vi "Measure Voltage.vi"(7 "Channel List (101:110)":string="101:110", 8 "error in (no error)":errorcluster, 10 "Sample Count":i32=1, 11 "VISA resource name":refnum<visa-resource-name>="COM15") -> (0 "error out":errorcluster, 2 "Voltage Data":dbl[](array[numeric])=[-0.0818253011], 3 "Voltage":dbl=-0.0818253011 format="%0.8f")   [LabVIEW 2015]
uses:
  <instrlib>/Keithley 27XX/Public/Data/Read Multiple Direct.vi
  <instrlib>/Keithley 27XX/Keithley 27XX.lvlib
panel:
  in  "Serial Configuration":T1={"Baud Rate (19200)"=19200, "Flow Control (1: XON/XOFF)"=1, "Termination Char (0:CR)"=0} {"Termination Char (0:CR)" items=["CR", "LF"]; "Flow Control (1: XON/XOFF)" items=["None", "XON/XOFF", "RTS/CTS (2701 Only)", "XON/XOFF & RTS/CTS (2701 Only)"]; "Baud Rate (19200)" items=["300"=300, "600"=600, "1200"=1200, "2400"=2400, "4800"=4800, "9600"=9600, "19.2k"=19200, "38.4k (2701 Only)"=38400, "57.6k (2701 Only)"=57600, "115.2k (2701 Only)"=115200]}
  in  "Timeout (5000 milliseconds)":u32=5000
  in  "Function (0: DC Voltage)":u16(ring) items=["DC Voltage", "AC Voltage", "DC Current", "AC Current", "Resistance", "Four-Wire Resistance", "Temperature (C)", "Frequency", "Period", "Continuity"]
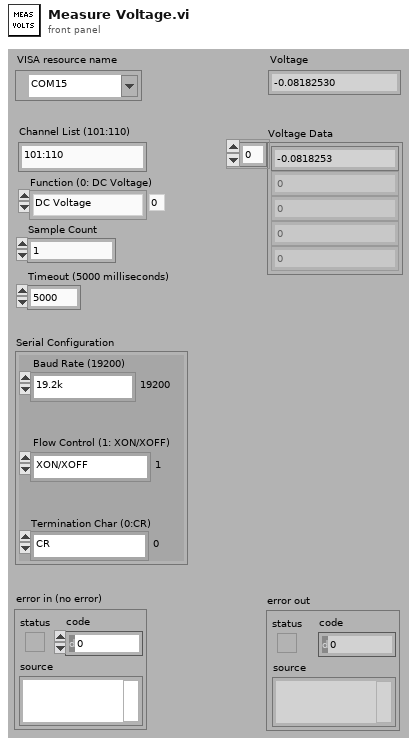
[diagram p1: front panel]
types:
  T1 = cluster{"Baud Rate (19200)":u32, "Flow Control (1: XON/XOFF)":u16, "Termination Char (0:CR)":u16}
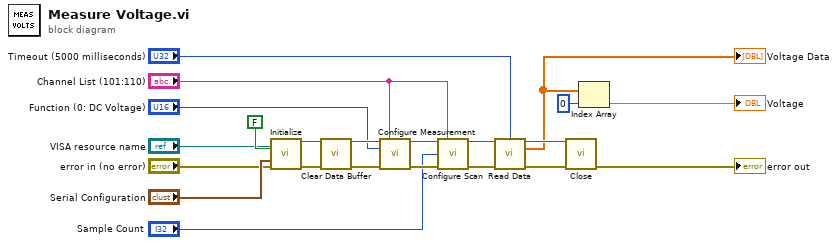
[diagram p0: block diagram]
diagram:
  n1 = call <instrlib>:"Initialize.vi"("VISA resource name"="VISA resource name", "ID Query? (T: Yes)"=FALSE, "Serial Configuration"="Serial Configuration", "error in (no error)"="error in (no error)") -> ("VISA resource name out"=w15:refnum<visa-resource-name>, "error out"=w16:errorcluster)  [unwired: 10 in]
  n2 = call <instrlib>:"Clear Data Buffer.vi"("VISA resource name"=w15, "error in (no error)"=w16) -> ("VISA resource name out"=w18:refnum<visa-resource-name>, "error out"=w17:errorcluster)  [unwired: 12 in]
  n3 = call <instrlib>:"Configure Measurement.vi"("VISA resource name"=w18, "Scan List (Empty)"="Channel List (101:110)", "Function (0: DC Voltage)"="Function (0: DC Voltage)", "error in (no error)"=w17) -> ("VISA resource name out"=w22:refnum<visa-resource-name>, "error out"=w19:errorcluster)  [unwired: 10 in]
  n4 = call <instrlib>:"Configure Scan.vi"("VISA resource name"=w22, "Channel List (101:110)"="Channel List (101:110)", "Sample Count (100)"="Sample Count", "error in (no error)"=w19) -> ("VISA resource name out"=w12:refnum<visa-resource-name>, "error out"=w13:errorcluster)  [unwired: 10 in]
  n5 = call-poly <instrlib>:"Read Data.vi"("VISA resource name"=w12, "Timeout (30000 milliseconds)"="Timeout (5000 milliseconds)", "error in (no error)"=w13) -> ("VISA resource name out"=w21:refnum<visa-resource-name>, "Measurement Data"=w7:dbl[], "error out"=w20:errorcluster)  [unwired: 7 in, 3 out]
  "Voltage Data" <- w7
  n6 = call <instrlib>:"Close.vi"("VISA resource name"=w21, "error in (no error)"=w20) -> ("error out"=→"error out":errorcluster)  [unwired: 13 in]
  n7 = Index Array(array=w7, index=0) -> (element=→"Voltage":dbl)
